vi "Configure Channel.vi"(8 "error in (no error)":errorcluster, 10 "DAQmx Task In":refnum<k21>, 11 "RTDChannel in":refnum<class "RTDChannel.lvclass">) -> (0 "error out":errorcluster, 2 "DAQmx Task":refnum<k21>)   [LabVIEW 2020, in "VolatusDAQConfig.lvlib" / "RTDChannel.lvclass"]
uses:
  RTDChannel.lvclass
  C:/dev/lv20CE/relink/lv-volatus/VolatusConfig/VolatusConfigElement/VolatusConfigElement.lvclass
  C:/dev/lv20CE/relink/lv-volatus/VolatusConfig/Channel/Channel.lvclass
  VolatusConfig/VolatusConfigElement/VolatusConfigElement.lvclass/VolatusConfigElement.ctl
  RTDChannel.lvclass/RTDChannel.ctl
  VolatusConfig/VolatusConfigElement/Element.vi
  VolatusConfig/VolatusConfigElement/Lookup Child by Name.vi
  VolatusConfig/Channel/Channel Config.lvclass
  lv-cdm/CDM-Config/Config Element/Lookup Child by Name.vi
  lv-cdm/CDM-Config/Config Element/Value (String).vi
  <vilib>/DAQmx/create/channels.llb/DAQmx Create Channel (AI-Temperature-RTD).vi
  VolatusConfig/VolatusConfigElement/VolatusConfigElement.lvclass
  C:/dev/lv20CE/relink/lv-volatus/VolatusDAQConfig/DAQmxChannel/DAQmxChannel.lvclass
  C:/dev/lv20CE/relink/lv-volatus/VolatusConfig/Channel/Channel Config.lvclass
  C:/dev/lv20CE/relink/lv-volatus/VolatusDAQConfig/RTDChannel/RTDChannel.lvclass
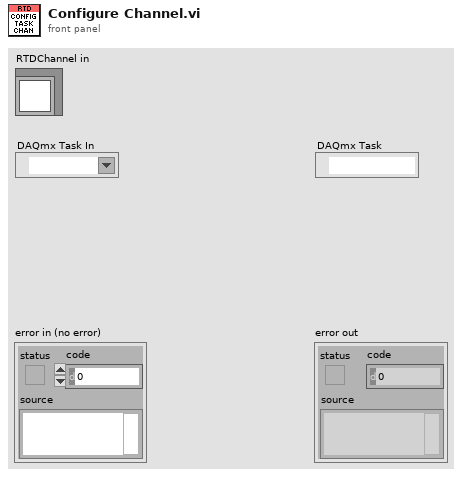
[diagram p1: front panel]
types:
  T1 = typedef "VolatusDAQConfig.lvlib/RTD Wiring.ctl" = enum16{"2-Wire", "3-Wire", "4-Wire"}
  T2 = typedef "VolatusDAQConfig.lvlib/Temperature Units.ctl" = enum16{"C", "F", "K", "R"}
  T3 = typedef "VolatusDAQConfig.lvlib/RTD Excitation.ctl" = enum16{"Internal", "External", "None"}
  T4 = typedef "VolatusDAQConfig.lvlib/RTD Type.ctl" = enum16{"Pt3750", "Pt3851", "Pt3911", "Pt3916", "Pt3920", "Pt3928", "Custom"}
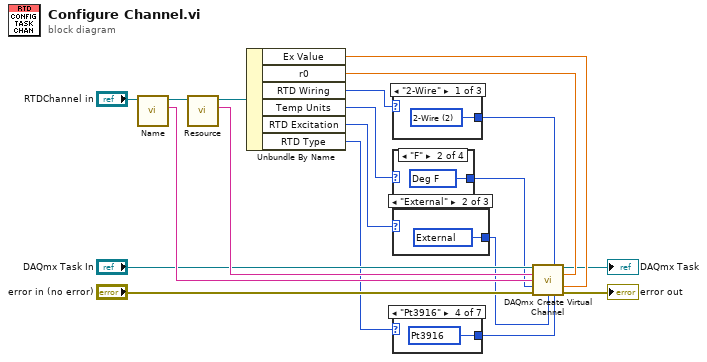
[diagram p0: block diagram]
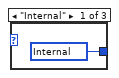
[diagram p2: hidden frame]
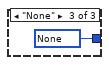
[diagram p3: hidden frame]
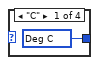
[diagram p4: hidden frame]
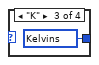
[diagram p5: hidden frame]
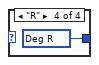
[diagram p6: hidden frame]
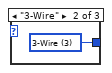
[diagram p7: hidden frame]
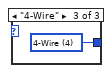
[diagram p8: hidden frame]
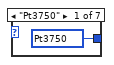
[diagram p9: hidden frame]
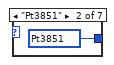
[diagram p10: hidden frame]
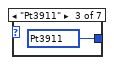
[diagram p11: hidden frame]
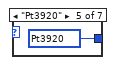
[diagram p12: hidden frame]
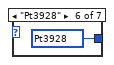
[diagram p13: hidden frame]
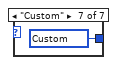
[diagram p14: hidden frame]
diagram:
  n1 = call "Name.vi"("VolatusConfigElement in"="RTDChannel in") -> ("Name"=w11:string, "VolatusConfigElement out"=w12:refnum<class "RTDChannel.lvclass">)  [unwired: 8 in, 1 out]
  n2 = call "Resource.vi"("Channel in"=w12) -> ("Resource"=w9:string, "Channel out"=w10:refnum<class "RTDChannel.lvclass">)  [unwired: 8 in, 1 out]
  n3 = Unbundle By Name(w10) -> ("Ex Value"=w16:dbl, "r0"=w15:dbl, "RTD Wiring"=w14:T1, "Temp Units"=w5:T2, "RTD Excitation"=w4:T3, "RTD Type"=w1:T4)
  n4 = case shown="\"2-Wire\"" w14 {
    tunnel: [w20 w21 w22] -> w13
    frame "2-Wire" {
      w20 = 2 items=["2-Wire"=2, "3-Wire"=3, "4-Wire"=4] ("resistance configuration")
    }
    frame "3-Wire" {
      w21 = 3 items=["2-Wire"=2, "3-Wire"=3, "4-Wire"=4] ("resistance configuration")
    }
    frame "4-Wire" {
      w22 = 4 items=["2-Wire"=2, "3-Wire"=3, "4-Wire"=4] ("resistance configuration")
    }
  }
  n5 = case shown="\"F\"" w5 {
    tunnel: [w23 w24 w25 w26] -> w6
    frame "C" {
      w23 = 10143 items=["Deg C"=10143, "Deg F"=10144, "Kelvins"=10325, "Deg R"=10145, "From Custom Scale"=10065] ("units")
    }
    frame "F" {
      w24 = 10144 items=["Deg C"=10143, "Deg F"=10144, "Kelvins"=10325, "Deg R"=10145, "From Custom Scale"=10065] ("units")
    }
    frame "K" {
      w25 = 10325 items=["Deg C"=10143, "Deg F"=10144, "Kelvins"=10325, "Deg R"=10145, "From Custom Scale"=10065] ("units")
    }
    frame "R" {
      w26 = 10145 items=["Deg C"=10143, "Deg F"=10144, "Kelvins"=10325, "Deg R"=10145, "From Custom Scale"=10065] ("units")
    }
  }
  n6 = case shown="\"External\"" w4 {
    tunnel: [w27 w28 w29] -> w3
    frame "Internal" {
      w27 = 10200 items=["Internal"=10200, "External"=10167, "None"=10230] ("current excitation source")
    }
    frame "External" {
      w28 = 10167 items=["Internal"=10200, "External"=10167, "None"=10230] ("current excitation source")
    }
    frame "None" {
      w29 = 10230 items=["Internal"=10200, "External"=10167, "None"=10230] ("current excitation source")
    }
  }
  n7 = case shown="\"Pt3916\"" w1 {
    tunnel: [w30 w31 w32 w33 w34 w35 w36] -> w2
    frame "Pt3750" {
      w30 = 12481 items=["Pt3750"=12481, "Pt3851"=10071, "Pt3911"=12482, "Pt3916"=10069, "Pt3920"=10053, "Pt3928"=12483, "Custom"=10137] ("rtd type")
    }
    frame "Pt3851" {
      w31 = 10071 items=["Pt3750"=12481, "Pt3851"=10071, "Pt3911"=12482, "Pt3916"=10069, "Pt3920"=10053, "Pt3928"=12483, "Custom"=10137] ("rtd type")
    }
    frame "Pt3911" {
      w32 = 12482 items=["Pt3750"=12481, "Pt3851"=10071, "Pt3911"=12482, "Pt3916"=10069, "Pt3920"=10053, "Pt3928"=12483, "Custom"=10137] ("rtd type")
    }
    frame "Pt3916" {
      w33 = 10069 items=["Pt3750"=12481, "Pt3851"=10071, "Pt3911"=12482, "Pt3916"=10069, "Pt3920"=10053, "Pt3928"=12483, "Custom"=10137] ("rtd type")
    }
    frame "Pt3920" {
      w34 = 10053 items=["Pt3750"=12481, "Pt3851"=10071, "Pt3911"=12482, "Pt3916"=10069, "Pt3920"=10053, "Pt3928"=12483, "Custom"=10137] ("rtd type")
    }
    frame "Pt3928" {
      w35 = 12483 items=["Pt3750"=12481, "Pt3851"=10071, "Pt3911"=12482, "Pt3916"=10069, "Pt3920"=10053, "Pt3928"=12483, "Custom"=10137] ("rtd type")
    }
    frame "Custom" {
      w36 = 10137 items=["Pt3750"=12481, "Pt3851"=10071, "Pt3911"=12482, "Pt3916"=10069, "Pt3920"=10053, "Pt3928"=12483, "Custom"=10137] ("rtd type")
    }
  }
  n8 = call-poly <vilib>:"DAQmx Create Virtual Channel.vi"("task in"="DAQmx Task In", "resistance configuration"=w13, "physical channels"=w9, "r0"=w15, "name to assign"=w11, "units"=w6, "current excitation value"=w16, "error in"="error in (no error)", "current excitation source"=w3, "rtd type"=w2) -> ("task out"=→"DAQmx Task":refnum<k21>, "error out"=→"error out":errorcluster)  [unwired: 4 in]
